vi "跨度核查数据发送 (子VI).vi"() -> (3 "超时退出":bool)   [LabVIEW 2016, in "数据传输系统-06.lvlib"]
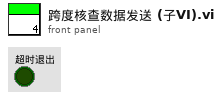
[diagram p1: front panel]
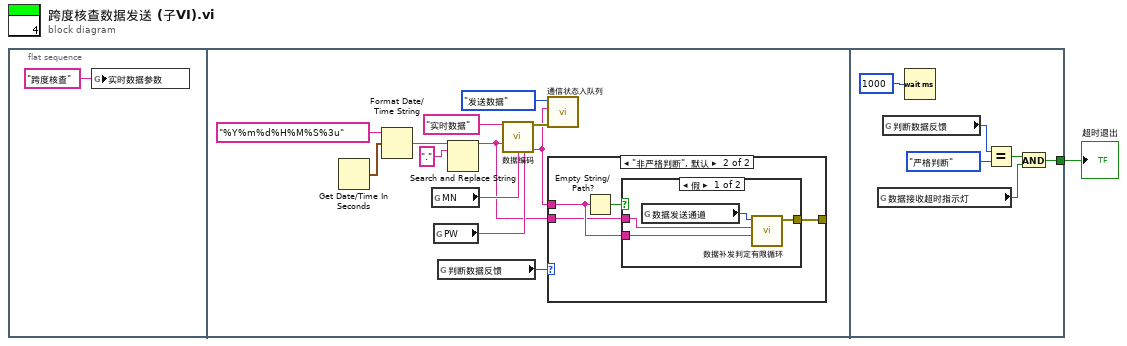
[diagram p0: block diagram]
diagram:
  n1 = flat-sequence {
    tunnel: [w23] -> w1
    frame #0 {
      n2 = global write "全局 实时数据参数.vi" "实时数据参数"("跨度核查") -> ()
    }
    frame #1 {
      n3 = Get Date/Time In Seconds() -> (seconds since 1Jan1904=w12:timestamp)
      n4 = Format Date/Time String(time format string (%c)="%Y%m%d%H%M%S%3u" ("时间格式字符串(%c)"), seconds (now)=w12) -> (date/time string=w13:string)  [unwired: 1 in]
      n5 = global read "断电保存全局.vi" "MN"() -> (w8:string)
      n6 = global read "断电保存全局.vi" "PW"() -> (w9:string)
      n7 = global read "断电保存全局.vi" "判断数据反馈"() -> (w6:enum16{"非严格判断", "严格判断", "不判断"})
      n8 = Search and Replace String(input string=w13, search string="." ("搜索字符串")) -> (result string=w5:string)  [unwired: 6 in, 3 out]
      n9 = call "数据编码.vi"("table输入"="实时数据" ("新元素/子数组"), "QN"=w5, "MN"=w8, "PW"=w9) -> ("错误常量"=w10:errorcluster, "通讯包字符串"=w3:string)  [unwired: 10 in]
      n10 = call "通信状态入队列.vi"("错误输入（无错误）"=w10, "发送报文"=w3, "枚举"=enum16{"打开连接", "发送数据", "读取数据", "数据处理", "关闭连接"}."发送数据") -> ()  [unwired: 8 in, 1 out]
      n11 = case shown="\"非严格判断\", 默认" w6 {
        tunnel: [_ w18] -> _
        tunnel: w3 -> [_ w17]
        tunnel: w5 -> [_ w16]
        frame "不判断" {
        }
        frame "非严格判断", Default {
          n12 = Empty String/Path?(string/path=w17) -> (empty?=w15:bool)
          n13 = case shown="假" w15 {
            tunnel: [w22 _] -> w18
            tunnel: w17 -> [w21 _]
            tunnel: w16 -> [w19 _]
            frame False {
              n14 = global read "断电保存全局.vi" "数据发送通道"() -> (w20:enum16{"TCP", "VISA"})
              n15 = call "数据补发判定有限循环.vi"("数据输入"=w21, "QN"=w19, "数据发送通道"=w20) -> ("error out"=w22:errorcluster)  [unwired: 8 in]
            }
            frame True {
            }
          }
        }
      }
    }
    frame #2 {
      n16 = global read "全局 数据发送重叠.vi" "数据接收超时指示灯"() -> (w24:bool)
      n17 = global read "断电保存全局.vi" "判断数据反馈"() -> (w27:enum16{"非严格判断", "严格判断", "不判断"})
      n18 = Wait (ms)(milliseconds to wait=u32 1000 ("等待时间（毫秒）")) -> ()  [unwired: 1 out]
      n19 = Equal?(x=w27, y=enum16{"非严格判断", "严格判断", "不判断"}."严格判断") -> (x = y?=w25:bool)
      n20 = And(x=w25, y=w24) -> (x .and. y?=w23:bool)
    }
  }
  "超时退出" <- w1
